vi "USB2XXXSPISlaveTest.vi"() -> ()   [LabVIEW 2010]
uses:
  PublicFiles/USB2XXX.dll
panel:
  out "Read Data(Hex)":string
  in  "stop 2":bool
  in  "Write Data(Hex)":string="11 22 33 44 55 66 77 88"
  in  "pConfig":T1
  in  "Channel Index":i32(ring) items=["SPI1_CS0", "SPI2_CS0"]
  in  "Device Index":i32(ring) items=["0", "1", "2", "3", "4", "5"]
  in  "Read":bool
  in  "Write":bool
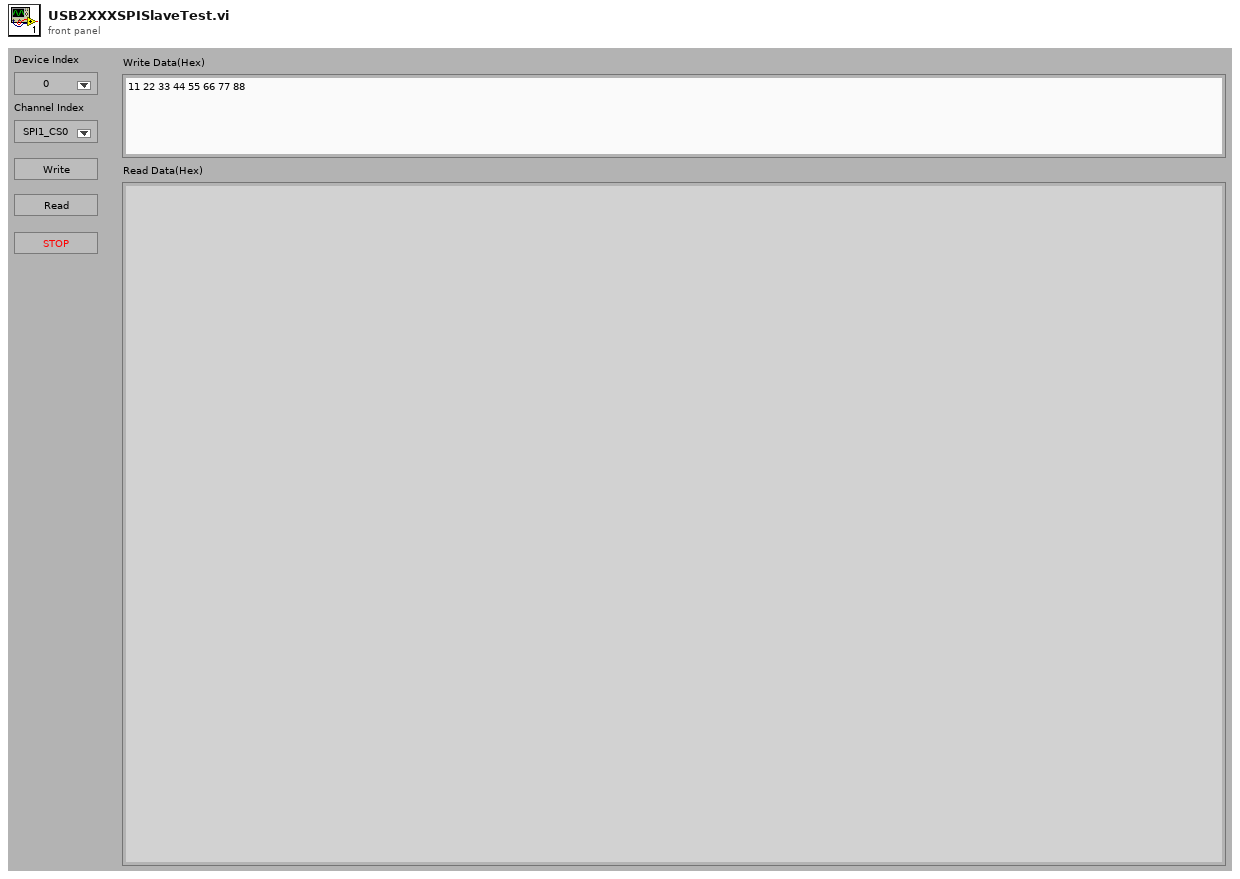
[diagram p1: front panel]
types:
  T1 = cluster{"Mode":i8, "Master":i8, "CPOL":i8, "CPHA":i8, "LSBFirst":i8, "SelPolarity":i8, "@dummy control@":i8, "@dummy control@":i8, "ClockSpeedHz":u32}
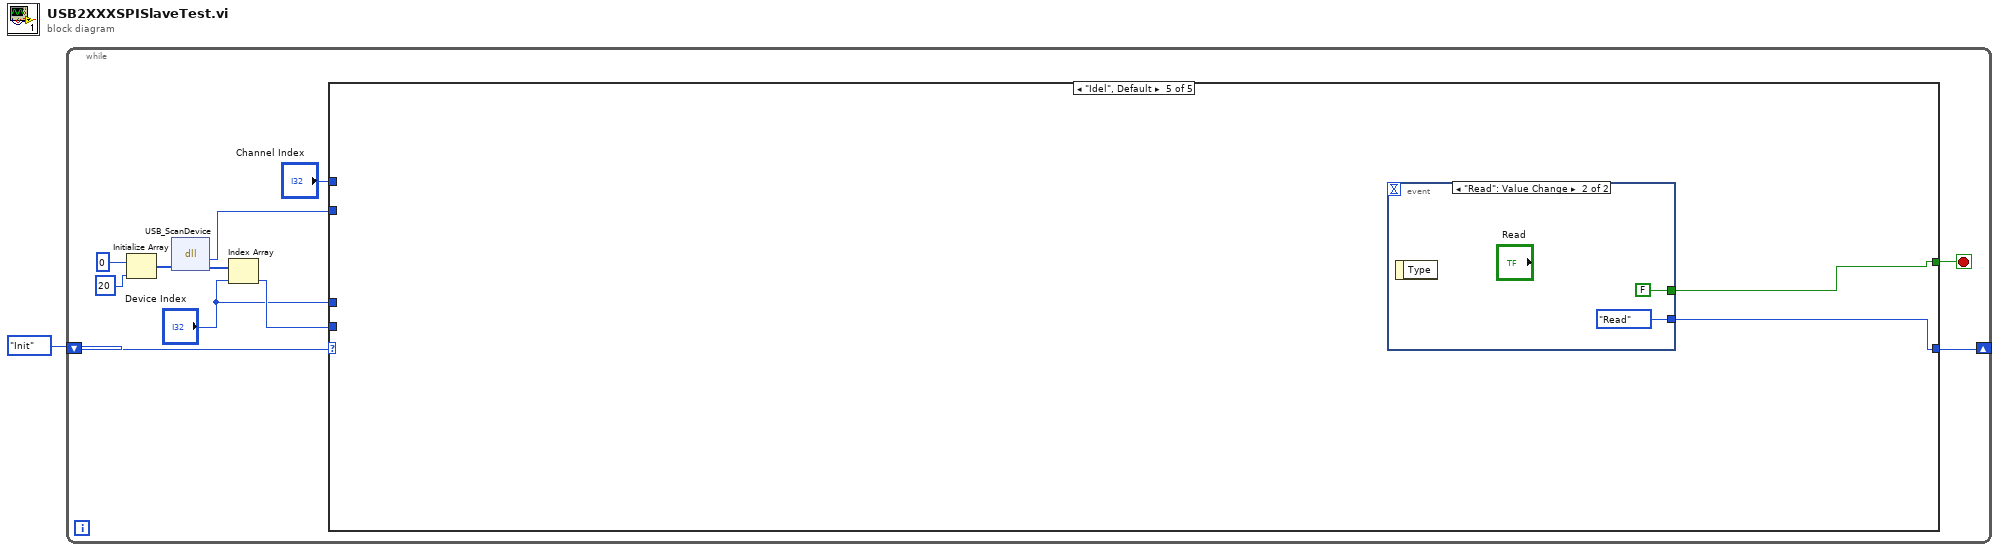
[diagram p0: block diagram]
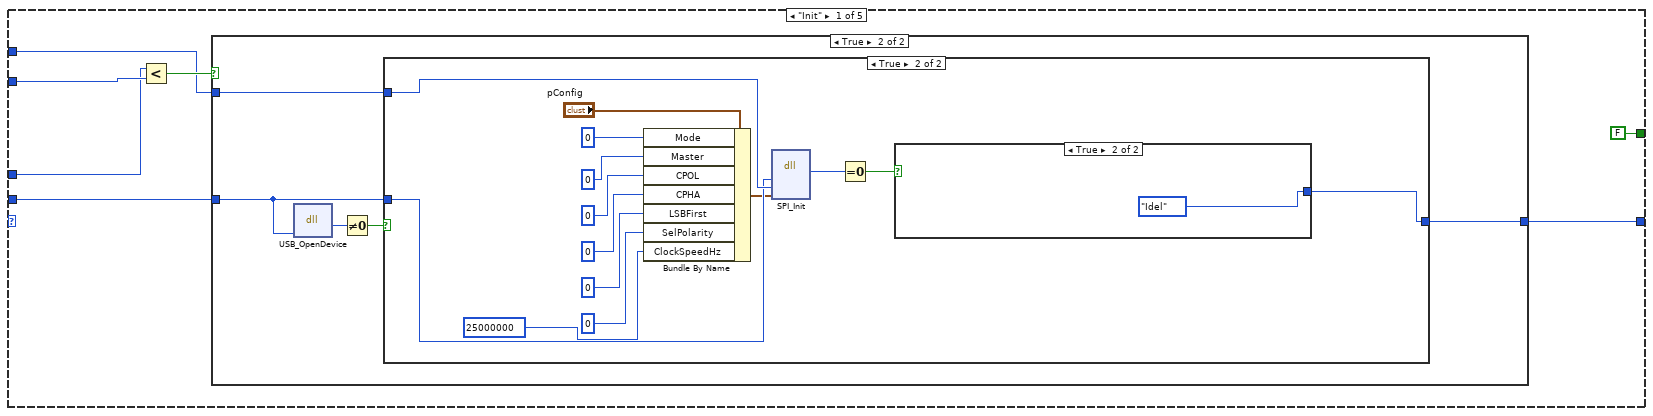
[diagram p2: hidden frame]
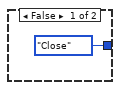
[diagram p3: hidden frame]
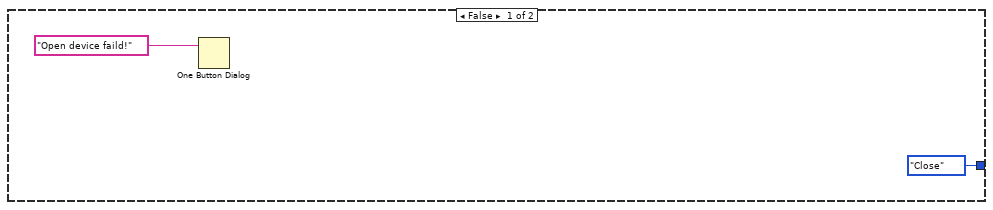
[diagram p4: hidden frame]
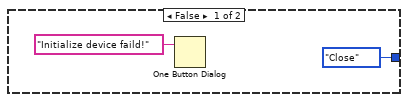
[diagram p5: hidden frame]
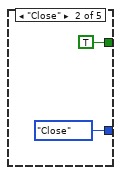
[diagram p6: hidden frame]
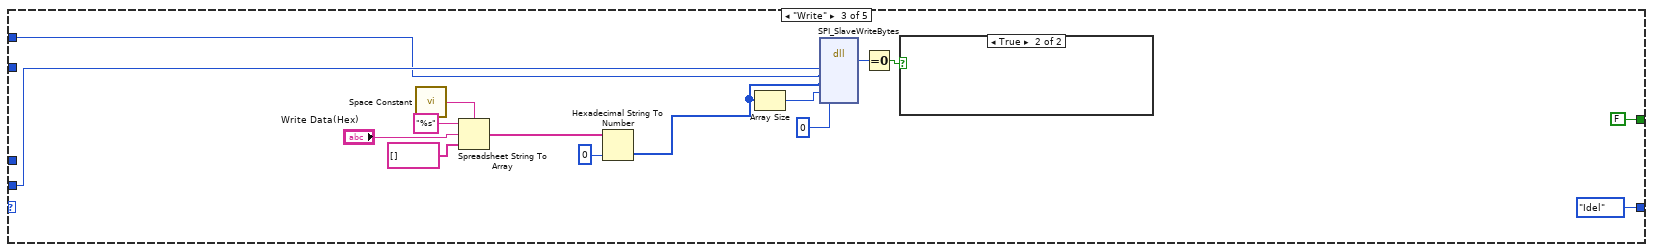
[diagram p7: hidden frame]
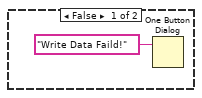
[diagram p8: hidden frame]
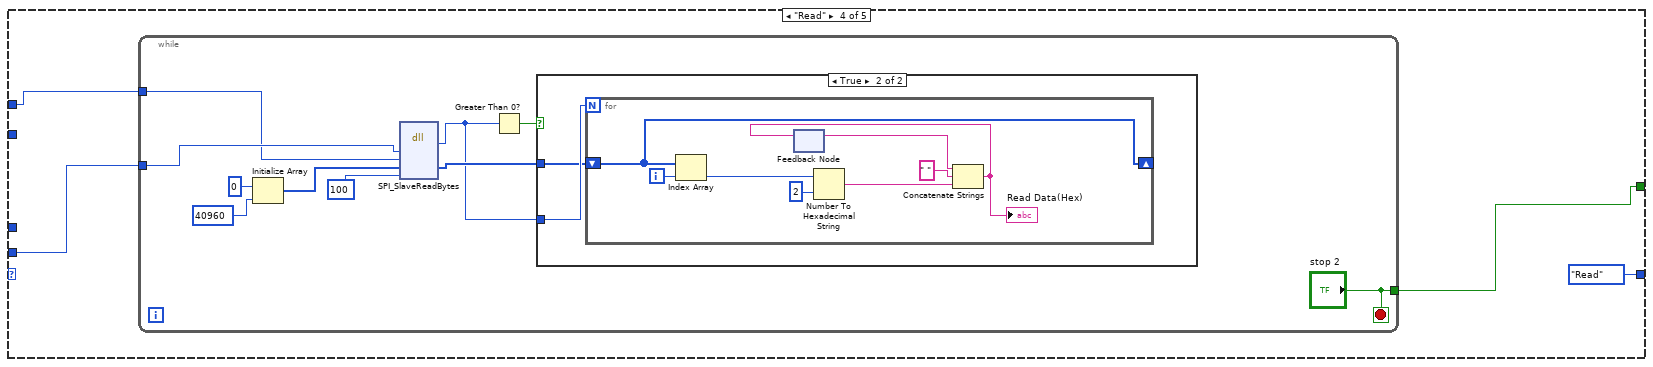
[diagram p9: hidden frame]
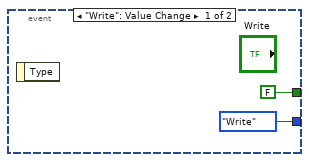
[diagram p11: hidden frame]
diagram:
  n1 = while {
    shift-right: [w11] -> _
    shift-left: enum16{"Init", "Write", "Read", "Idel", "Close"}."Init" ("Enum") -> [w12]
    stop <- w9 stop-if-true
    n2 = Initialize Array(0, 20 ("dimension size")) -> (w8:i32[])
    n3 = dll-call lib="F:/OtherWork/STM32/USB2XXX_Example/trunk/Labview/PublicFiles/USB2XXX.*" fn="USB_ScanDevice"("pDevNum"=w8) -> ("return type"=w4:i32, "pDevNum"=w6:i32[])  [unwired: 3 in, 2 out]
    n4 = Index Array(array=w6, index="Device Index") -> (element=w5:i32)
    n5 = case shown="\"Idel\", Default" w12 {
      tunnel: [w18 enum16{"Init", "Write", "Read", "Idel", "Close"}."Close" ("Enum") enum16{"Init", "Write", "Read", "Idel", "Close"}."Idel" ("Enum") enum16{"Init", "Write", "Read", "Idel", "Close"}."Read" ("Enum") w88] -> w11
      tunnel: w5 -> [w15 _ w52 w64 _]
      tunnel: "Channel Index" -> [w17 _ w51 w63 _]
      tunnel: [FALSE TRUE FALSE w65 w87] -> w9
      tunnel: w4 -> [w14 _ _ _ _]
      tunnel: "Device Index" -> [w13 _ _ _ _]
      frame "Init" {
        n6 = Less?(x=w13, y=w14) -> (x < y?=w19:bool)
        n7 = case shown="True" w19 {
          tunnel: w15 -> [_ w21]
          tunnel: w17 -> [_ w23]
          tunnel: [enum16{"Init", "Write", "Read", "Idel", "Close"}."Close" ("Enum") w22] -> w18
          frame False {
          }
          frame True {
            n8 = dll-call lib="F:/OtherWork/STM32/USB2XXX_Example/trunk/Labview/PublicFiles/USB2XXX.*" fn="USB_OpenDevice"("DevIndex"=w21) -> (w25:u8)  [unwired: 4 in, 2 out]
            n9 = Not Equal To 0?(x=w25) -> (x != 0?=w24:bool)
            n10 = case shown="True" w24 {
              tunnel: w23 -> [_ w39]
              tunnel: w21 -> [_ w38]
              tunnel: [enum16{"Init", "Write", "Read", "Idel", "Close"}."Close" ("Enum") w40] -> w22
              frame False {
                n11 = One Button Dialog(message="Open device faild!") -> ()  [unwired: 1 in, 1 out]
              }
              frame True {
                n12 = Bundle By Name(cluster="pConfig", "Mode"=i8 0, "Master"=i8 0, "CPOL"=i8 0, "CPHA"=i8 0, "LSBFirst"=i8 0, "SelPolarity"=i8 0, "ClockSpeedHz"=u32 25000000) -> (w37:T1)
                n13 = dll-call lib="F:/OtherWork/STM32/USB2XXX_Example/trunk/Labview/PublicFiles/USB2XXX.*" fn="SPI_Init"("DevIndex"=w38, "SPIIndex"=w39, "pConfig"=w37) -> (w36:i32)  [unwired: 6 in, 2 out]
                n14 = Equal To 0?(x=w36) -> (x = 0?=w41:bool)
                n15 = case shown="True" w41 {
                  tunnel: [enum16{"Init", "Write", "Read", "Idel", "Close"}."Close" ("Enum") enum16{"Init", "Write", "Read", "Idel", "Close"}."Idel" ("Enum")] -> w40
                  frame False {
                    n16 = One Button Dialog(message="Initialize device faild!") -> ()  [unwired: 1 in, 1 out]
                  }
                  frame True {
                  }
                }
              }
            }
          }
        }
      }
      frame "Close" {
      }
      frame "Write" {
        n17 = call <vilib>:"Space Constant.vi"() -> ("String"=w57:string)
        n18 = Spreadsheet String To Array(delimiter (Tab)=w57, format string="%s", spreadsheet string="Write Data(Hex)", array type (2D Dbl)=string[] []) -> (array=w54:string[])
        n19 = Hexadecimal String To Number(string=w54, default (0uL)=u8 0 ("default (0 U32)")) -> (number=w50:u8[])  [unwired: 1 in, 1 out]
        n20 = Array Size(array=w50) -> (size(s)=w48:i32)
        n21 = dll-call lib="F:/OtherWork/STM32/USB2XXX_Example/trunk/Labview/PublicFiles/USB2XXX.*" fn="SPI_SlaveWriteBytes"("DevHandle"=w52, "SPIIndex"=w51, "pWriteData"=w50, "WriteLen"=w48, "TimeOutMs"=0) -> (w49:i32)  [unwired: 8 in, 2 out]
        n22 = Equal To 0?(x=w49) -> (x = 0?=w59:bool)
        n23 = case shown="True" w59 {
          frame False {
            n24 = One Button Dialog(message="Write Data Faild!") -> ()  [unwired: 1 in, 1 out]
          }
          frame True {
          }
        }
      }
      frame "Read" {
        n25 = while {
          tunnel: ["stop 2"] -> w65
          tunnel: w64 -> [w68]
          tunnel: w63 -> [w67]
          stop <- "stop 2" stop-if-true
          n26 = Initialize Array(u8 0 ("element"), 40960 ("element")) -> (w73:u8[])
          n27 = dll-call lib="F:/OtherWork/STM32/USB2XXX_Example/trunk/Labview/PublicFiles/USB2XXX.*" fn="SPI_SlaveReadBytes"("DevHandle"=w68, "SPIIndex"=w67, "pReadData"=w73, "TimeOutMs"=100) -> (w69:i32, "pReadData"=w70:u8[])  [unwired: 6 in, 2 out]
          n28 = Greater Than 0?(x=w69) -> (x > 0?=w74:bool)
          n29 = case shown="True" w74 {
            tunnel: w69 -> [_ w78]
            tunnel: w70 -> [_ w77]
            frame False {
            }
            frame True {
              n30 = for {
                N: w78 -> [_]
                shift-right: [w79] -> _
                shift-left: w77 -> [w79]
                i -> [w86]
                n31 = Index Array(array=w79, index=w86) -> (element=w85:u8)
                n32 = feedback #1() -> (w83:string)  [unwired: 1 in]
                n33 = Number To Hexadecimal String(1:i16 2 ("width (-)"), 2:w85) -> (0:w81:string)
                n34 = Concatenate Strings(w83, " " ("string"), w81) -> (w80:string)
                "Read Data(Hex)" <- w80
                n35 = feedback-in #1(w80) -> ()
              }
            }
          }
        }
      }
      frame "Idel", Default {
        n36 = event shown="[1] \"Read\": Value Change" {
          selector: _ -> [_ _]
          dyn-events: _ -> [_ _]
          timeout: _ -> [_ _]
          tunnel: [FALSE FALSE] -> w87
          tunnel: [enum16{"Init", "Write", "Read", "Idel", "Close"}."Write" ("Enum") enum16{"Init", "Write", "Read", "Idel", "Close"}."Read" ("Enum")] -> w88
          event "Write": Value Change {
            n37 = event-data() -> ()  [unwired: 1 in, 1 out]
          }
          event "Read": Value Change {
            n38 = event-data() -> ()  [unwired: 1 in, 1 out]
          }
        }
      }
    }
  }
